vi "setControlValues.vi"(8 "error in (no error)":errorcluster, 10 "Controls - Value":string[][](table), 11 "uiControlsMgr in":refnum<class "uiControlsMgr.lvclass">) -> (0 "error out":errorcluster, 3 "uiControlsMgr out":refnum<class "uiControlsMgr.lvclass">)   [LabVIEW 2020, in "uiControlsMgr.lvclass"]
uses:
  uiControlsMgr.lvclass
  uiControlsMgr.lvclass/uiControlsMgr.ctl
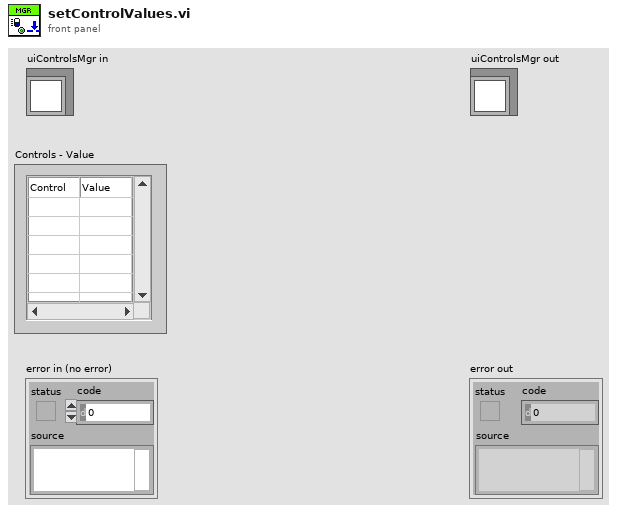
[diagram p1: front panel]
types:
  T1 = map{string, cluster{"Caption":string, "Ctl Refnum":refnum<vi>}}
  T2 = cluster{"Caption":string, "Ctl Refnum":refnum<vi>}
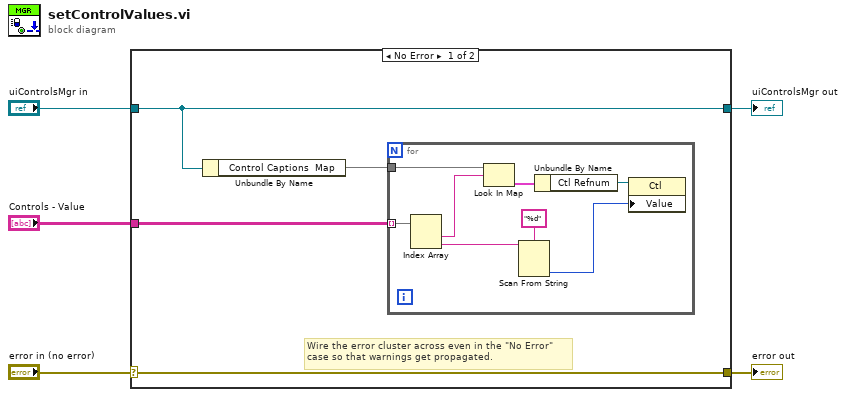
[diagram p0: block diagram]
diagram:
  n1 = case shown="No Error" "error in (no error)" {
    selector: "error in (no error)" -> [w9 w19]
    tunnel: [w9 w19] -> w4
    tunnel: [w7 w18] -> w2
    tunnel: "uiControlsMgr in" -> [w7 w18]
    tunnel: "Controls - Value" -> [w6 _]
    frame No Error {
      # "Wire the error cluster across even in the \"No Error\"\ncase so that warnings get propagated."
      n2 = Unbundle By Name(w7) -> ("Control Captions  Map"=w8:T1)
      n3 = for {
        tunnel: w8 -> [w17]
        tunnel: w6 -> [w16] mode=indexing
        n4 = Index Array(array=w16) -> (element #1=w15:string, element #2=w11:string)  [unwired: 2 in]
        n5 = Look In Map(map=w17, key=w15) -> (value=w14:T2)  [unwired: 1 in, 1 out]
        n6 = Scan From String(format string="%d", input string=w11) -> (output 1=w12:i32)  [unwired: 3 in, 3 out]
        n7 = Unbundle By Name(w14) -> ("Ctl Refnum"=w13:refnum<vi>)
        n8 = property class="Ctl"(reference=w13, "Value"=w12) -> ()  [unwired: 1 in, 2 out]
      }
    }
    frame Error {
    }
  }
  "error out" <- w4
  "uiControlsMgr out" <- w2
